vi "SweepMatrix.vi"(3 "Time Stamp":timestamp, 4 "From V2 to V1":bool=TRUE, 5 "From 0 to V1 and V2 to 0":bool, 6 "Play Button":bool, 7 "Rate w/o measure, V/min":dbl=30.0 min=0.0 max=1.0 step=0.01 format="%.4f", 8 "Custom Folder":string, 9 "Sweep rate, V/min":dbl=3.0 min=0.0 max=1.0 step=0.01 format="%.4f", 10 "V2 (V)":dbl=1.0 min=-4.0 max=4.0 step=0.1 format="%.4f", 11 "V1 (V)":dbl=-1.0 min=-4.0 max=4.0 step=0.1 format="%.4f") -> ()   [LabVIEW 2015]
uses:
  <vilib>/Utility/file.llb/Read From Spreadsheet File (DBL).vi
panel:
  out "ArraySens":i8[](array[numeric])
  out "ArrayOsc":dbl[](array[numeric])
  in  "From V2 to 0":bool
  in  "From V1 to V2":bool=TRUE
  out "# of configurations":i8
  out "Large Array":bool[][][](array[boolean])
  out "Contact configuration file (*.conf)":path
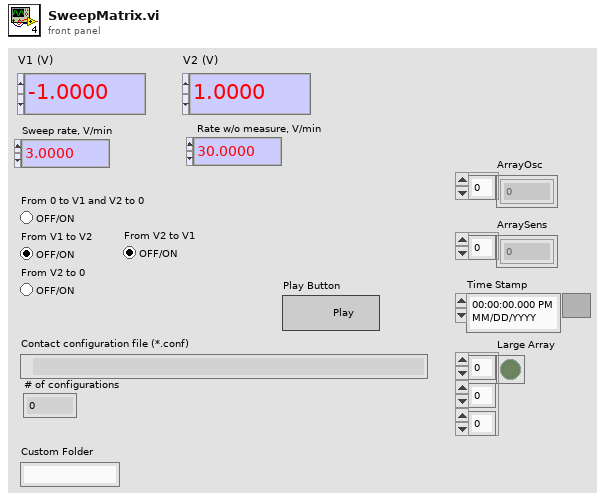
[diagram p1: front panel]
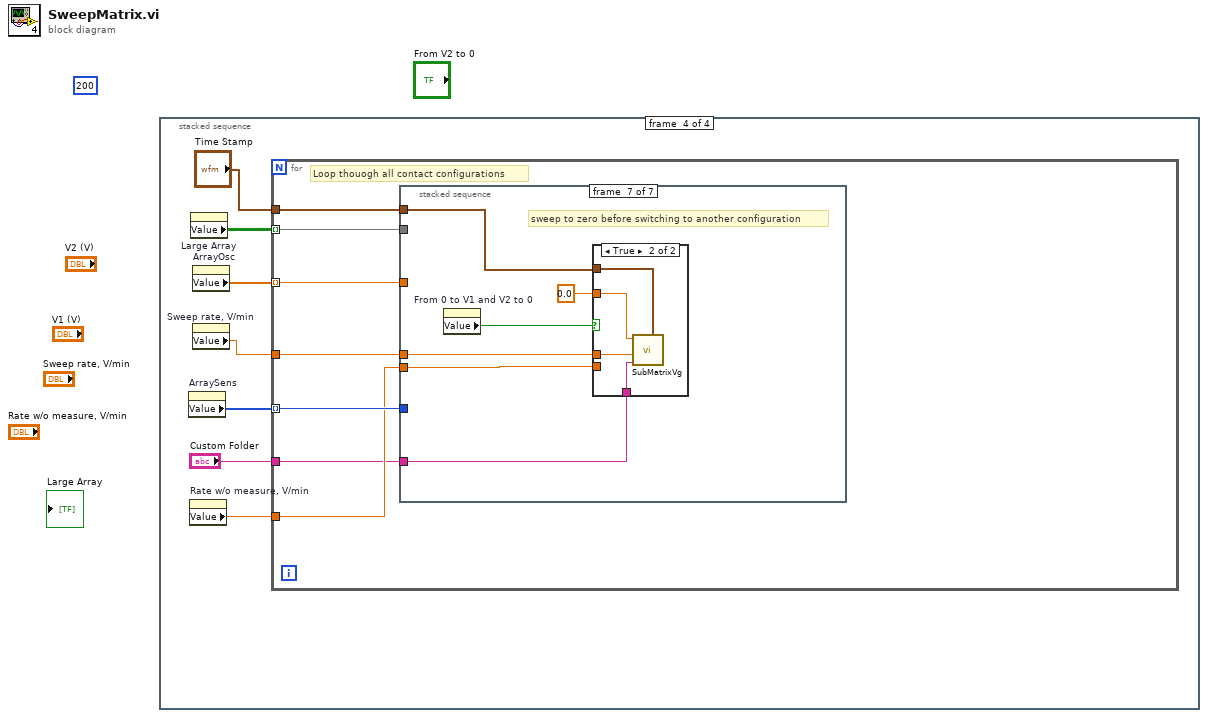
[diagram p0: block diagram]
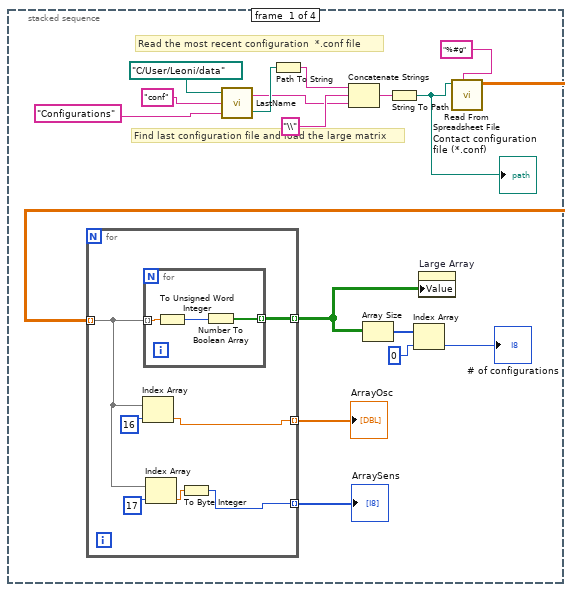
[diagram p2: hidden frame]
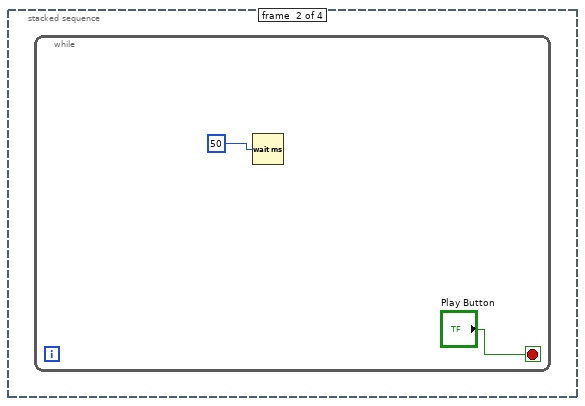
[diagram p3: hidden frame]
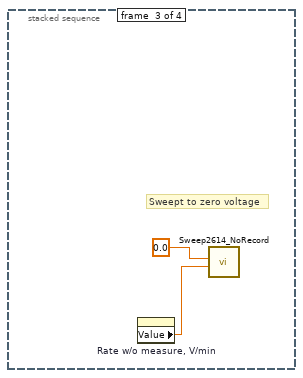
[diagram p4: hidden frame]
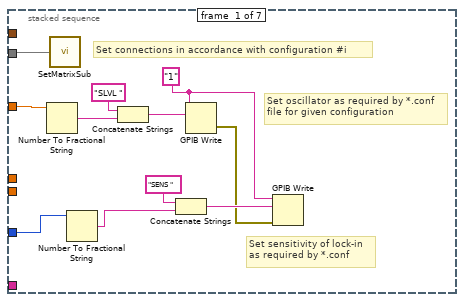
[diagram p5: hidden frame]
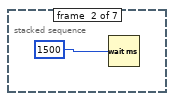
[diagram p6: hidden frame]
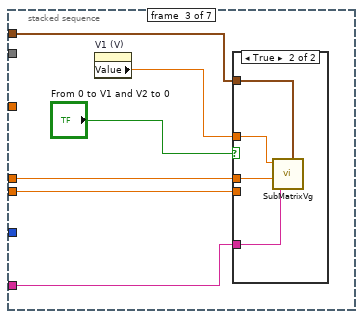
[diagram p7: hidden frame]
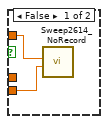
[diagram p8: hidden frame]
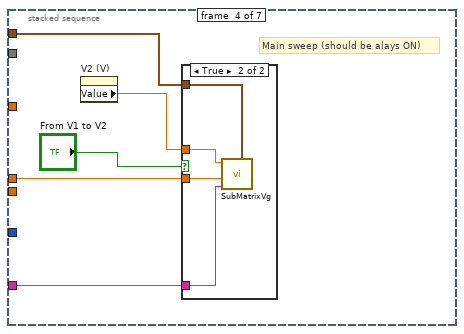
[diagram p9: hidden frame]
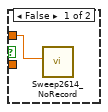
[diagram p10: hidden frame]
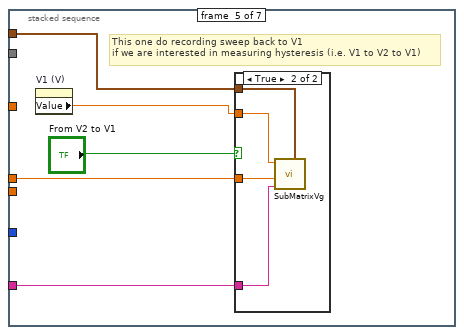
[diagram p11: hidden frame]
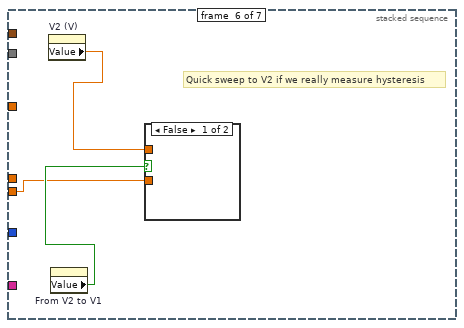
[diagram p13: hidden frame]
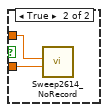
[diagram p14: hidden frame]
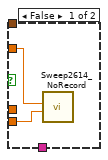
[diagram p15: hidden frame]
diagram:
  (unwired) 200
  n1 = stacked-sequence {
    frame #0 {
      # "Read the most recent configuration  *.conf file"
      # "Find last configuration file and load the large matrix"
      n2 = call "LastName.vi"("Custom Folder"="Configurations", "Extention"="conf", "User Data Folder"=path "C:/User/Leoni/data") -> ("created path"=w13:path, "String"=w12:string)
      n3 = Path To String(path=w13) -> (string=w17:string)
      n4 = Concatenate Strings(w17, "\\", w12) -> (w15:string)
      n5 = String To Path(string=w15) -> (path=w3:path)
      "Contact configuration file (*.conf)" <- w3
      n6 = call-poly <vilib>:"Read From Spreadsheet File.vi"("format (%.3f)"="%#g", "file path (dialog if empty)"=w3) -> ("all rows"=w8:dbl[][])  [unwired: 5 in, 4 out]
      n7 = for {
        tunnel: w8 -> [w20] mode=indexing
        tunnel: [w24] -> w5 mode=indexing
        tunnel: [w19] -> w2 mode=indexing
        tunnel: [w18] -> w1 mode=indexing
        n8 = Index Array(array=w20, index=16) -> (element=w19:dbl)
        n9 = for {
          tunnel: w20 -> [w27] mode=indexing
          tunnel: [w25] -> w24 mode=indexing
          n10 = To Unsigned Word Integer(number=w27) -> (unsigned 16bit integer=w26:u16)
          n11 = Number To Boolean Array(number=w26) -> (Boolean array=w25:bool[])
        }
        n12 = Index Array(array=w20, index=17) -> (element=w21:dbl)
        n13 = To Byte Integer(number=w21) -> (8bit integer=w18:i8)
      }
      "ArrayOsc" <- w2
      "ArraySens" <- w1
      n14 = Array Size(array=w5) -> (size(s)=w7:i32[])
      n15 = Index Array(array=w7, index=0) -> (element=→"# of configurations":i32)
      n16 = property on="Large Array" class="Arr (strict)"("Value"=w5) -> ()  [unwired: 2 in, 2 out]
    }
    frame #1 {
      n17 = while {
        stop <- "Play Button" stop-if-true
        n18 = Wait (ms)(milliseconds to wait=50) -> ()  [unwired: 1 out]
      }
    }
    frame #2 {
      # "Sweept to zero voltage"
      n19 = property on="Rate w/o measure, V/min" class="DigNum (strict)"() -> ("Value"=w30:dbl)  [unwired: 2 in, 2 out]
      n20 = call "Sweep2614_NoRecord.vi"("Rate (V/min)"=w30, "Vfinal (V)"=0.0) -> ()  [unwired: 2 in, 1 out]
    }
    frame #3 {
      n21 = property on="ArraySens" class="Arr (strict)"() -> ("Value"=w36:i8[])  [unwired: 2 in, 2 out]
      n22 = property on="Rate w/o measure, V/min" class="DigNum (strict)"() -> ("Value"=w35:dbl)  [unwired: 2 in, 2 out]
      n23 = property on="Large Array" class="Arr (strict)"() -> ("Value"=w38:bool[][][])  [unwired: 2 in, 2 out]
      n24 = property on="ArrayOsc" class="Arr (strict)"() -> ("Value"=w37:dbl[])  [unwired: 2 in, 2 out]
      n25 = property on="Sweep rate, V/min" class="DigNum (strict)"() -> ("Value"=w33:dbl)  [unwired: 2 in, 2 out]
      n26 = for {
        tunnel: w38 -> [w45] mode=indexing
        tunnel: w37 -> [w44] mode=indexing
        tunnel: w36 -> [w43] mode=indexing
        tunnel: w35 -> [w42]
        tunnel: "Custom Folder" -> [w41]
        tunnel: w33 -> [w40]
        tunnel: "Time Stamp" -> [w39]
        # "Loop thouogh all contact configurations"
        n27 = stacked-sequence {
          tunnel: w45 -> [w56 _ _ _ _ _ _]
          tunnel: w44 -> [w52 _ _ _ _ _ _]
          tunnel: w43 -> [w47 _ _ _ _ _ _]
          tunnel: w42 -> [_ _ w61 _ _ w89 w97]
          tunnel: w41 -> [_ _ w60 w72 w84 _ w95]
          tunnel: w40 -> [_ _ w59 w71 w83 _ w96]
          tunnel: w39 -> [_ _ w58 w70 w80 _ w94]
          frame #0 {
            w48 = "1"
            # "Set sensitivity of lock-in\nas required by *.conf"
            # "Set oscillator as required by *.conf\nfile for given configuration"
            # "Set connections in accordance with configuration #i"
            n28 = Number To Fractional String(number=w52) -> (F-format string=w55:string)  [unwired: 3 in]
            n29 = call "SetMatrixSub.vi"("Array"=w56) -> ()  [unwired: 1 in]
            n30 = Number To Fractional String(number=w47) -> (F-format string=w51:string)  [unwired: 3 in]
            n31 = Concatenate Strings("SLVL ", w55) -> (w54:string)
            n32 = Concatenate Strings("SENS ", w51) -> (w50:string)
            n33 = GPIB Write(0:w48, 1:w54) -> (6:w46:errorcluster)  [unwired: 3 in, 1 out]
            n34 = GPIB Write(0:w48, 1:w50, 3:w46) -> ()  [unwired: 2 in, 2 out]
          }
          frame #1 {
            n35 = Wait (ms)(milliseconds to wait=1500) -> ()  [unwired: 1 out]
          }
          frame #2 {
            n36 = property on="V1 (V)" class="DigNum (strict)"() -> ("Value"=w63:dbl)  [unwired: 2 in, 2 out]
            n37 = case shown="True" "From 0 to V1 and V2 to 0" {
              tunnel: w63 -> [w65 w69]
              tunnel: w61 -> [w64 _]
              tunnel: w60 -> [_ w68]
              tunnel: w59 -> [_ w67]
              tunnel: w58 -> [_ w66]
              frame False {
                n38 = call "Sweep2614_NoRecord.vi"("Rate (V/min)"=w64, "Vfinal (V)"=w65) -> ()  [unwired: 2 in, 1 out]
              }
              frame True {
                n39 = call "SubMatrixVg.vi"("Target Voltage, V"=w69, "Sweep rate, V/min"=w67, "Custom Folder"=w68, "Time Stamp"=w66) -> ()  [unwired: 6 in]
              }
            }
          }
          frame #3 {
            # "Main sweep (should be alays ON)"
            n40 = property on="V2 (V)" class="DigNum (strict)"() -> ("Value"=w74:dbl)  [unwired: 2 in, 2 out]
            n41 = case shown="True" "From V1 to V2" {
              tunnel: w74 -> [w75 w79]
              tunnel: w71 -> [_ w78]
              tunnel: w72 -> [_ w77]
              tunnel: w70 -> [_ w76]
              frame False {
                n42 = call "Sweep2614_NoRecord.vi"("Vfinal (V)"=w75) -> ()  [unwired: 3 in, 1 out]
              }
              frame True {
                n43 = call "SubMatrixVg.vi"("Target Voltage, V"=w79, "Sweep rate, V/min"=w78, "Custom Folder"=w77, "Time Stamp"=w76) -> ()  [unwired: 6 in]
              }
            }
          }
          frame #4 {
            # "This one do recording sweep back to V1\nif we are interested in measuring hysteresis (i.e. V1 to V2 to V1)"
            n44 = property on="V1 (V)" class="DigNum (strict)"() -> ("Value"=w81:dbl)  [unwired: 2 in, 2 out]
            n45 = case shown="True" "From V2 to V1" {
              tunnel: w81 -> [_ w88]
              tunnel: w83 -> [_ w87]
              tunnel: w84 -> [_ w86]
              tunnel: w80 -> [_ w85]
              frame False {
              }
              frame True {
                n46 = call "SubMatrixVg.vi"("Target Voltage, V"=w88, "Sweep rate, V/min"=w87, "Custom Folder"=w86, "Time Stamp"=w85) -> ()  [unwired: 6 in]
              }
            }
          }
          frame #5 {
            # "Quick sweep to V2 if we really measure hysteresis"
            n47 = property on="V2 (V)" class="DigNum (strict)"() -> ("Value"=w90:dbl)  [unwired: 2 in, 2 out]
            n48 = property on="From V2 to V1" class="Bool (strict)"() -> ("Value"=w91:bool)  [unwired: 2 in, 2 out]
            n49 = case shown="False" w91 {
              tunnel: w90 -> [_ w93]
              tunnel: w89 -> [_ w92]
              frame False {
              }
              frame True {
                n50 = call "Sweep2614_NoRecord.vi"("Rate (V/min)"=w92, "Vfinal (V)"=w93) -> ()  [unwired: 2 in, 1 out]
              }
            }
          }
          frame #6 {
            # "sweep to zero before switching to another configuration"
            n51 = property on="From 0 to V1 and V2 to 0" class="Bool (strict)"() -> ("Value"=w98:bool)  [unwired: 2 in, 2 out]
            n52 = case shown="True" w98 {
              tunnel: 0.0 -> [w101 w105]
              tunnel: w97 -> [w100 _]
              tunnel: w96 -> [_ w104]
              tunnel: w95 -> [_ w103]
              tunnel: w94 -> [_ w102]
              frame False {
                n53 = call "Sweep2614_NoRecord.vi"("Rate (V/min)"=w100, "Vfinal (V)"=w101) -> ()  [unwired: 2 in, 1 out]
              }
              frame True {
                n54 = call "SubMatrixVg.vi"("Target Voltage, V"=w105, "Sweep rate, V/min"=w104, "Custom Folder"=w103, "Time Stamp"=w102) -> ()  [unwired: 6 in]
              }
            }
          }
        }
      }
    }
  }
